vi "Global Oxford.vi"() -> ()   [LabVIEW 2022 SP3]
panel:
  in  "IPS Info.":T1 {"Status" items=["Stable", "Tracking"]; "Mode" items=["Persistent", "Driven"]}
  in  "IPS Addr":refnum<visa-resource-name>
  in  "VTI Info.":T2 {"Status" items=["Stable", "Tracking"]}
  in  "VTI Addr":refnum<visa-resource-name>
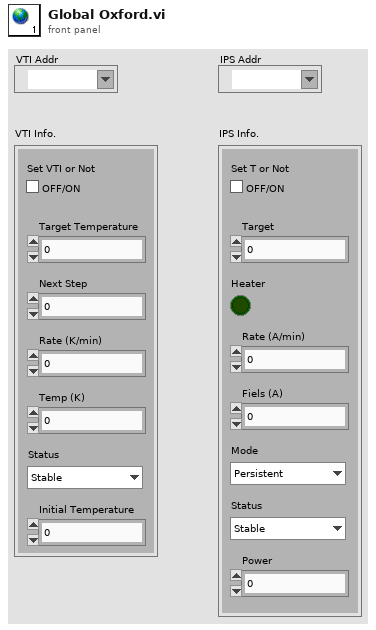
[diagram p1: front panel]
types:
  T1 = cluster{"Set T or Not":bool, "Rate (A/min)":dbl, "Target":dbl, "Fiels (A)":dbl, "Mode":u16, "Power":dbl, "Heater":bool, "Status":u16}
  T2 = cluster{"Set VTI or Not":bool, "Rate (K/min)":dbl, "Target Temperature":dbl, "Next Step":dbl, "Temp (K)":dbl, "Status":u16, "Initial Temperature":dbl}
diagram:
